vi "ping全局.vi"() -> ()   [LabVIEW 2016]
panel:
  out "配置文件 path":path
  out "ping":bool
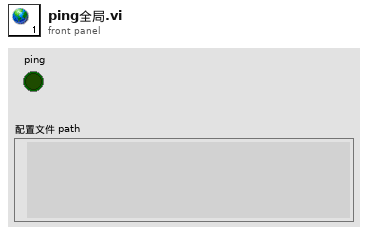
[diagram p1: front panel]
diagram:
